vi "CMD_TRANSFORMG2L.vi"(8 "error in (no error)":errorcluster, 10 "Arguments":string[](array[string]), 11 "gScript Interpreter in":refnum<class "gScript Interpreter.lvclass">) -> (0 "error out":errorcluster, 3 "gScript Interpreter out":refnum<class "gScript Interpreter.lvclass">)   [LabVIEW 2017, in "gScript Interpreter.lvclass"]
uses:
  gScript Interpreter.lvclass
  Shared Components/Utils/Type Definitions/Position_Orientation.ctl
  Shared Components/Vec3d Class/Vec3d.lvclass
  Shared Components/Orient3d Class/Orient3d.lvclass
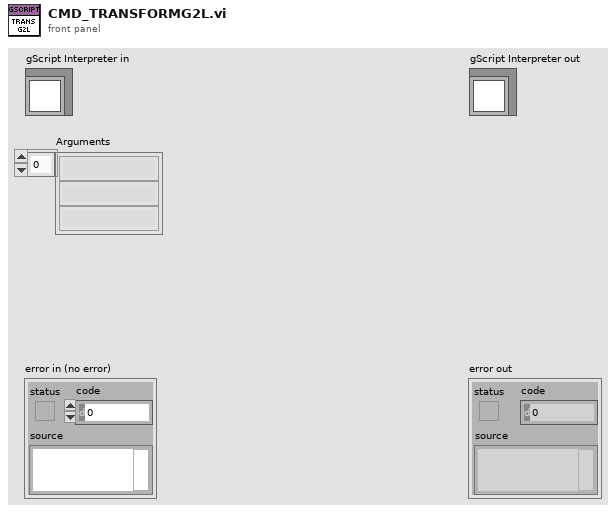
[diagram p1: front panel]
types:
  T1 = typedef "Position_Orientation.ctl" = cluster{"Center":refnum<class "Vec3d.lvclass">, "Orientation":refnum<class "Orient3d.lvclass">}
  T2 = typedef "Memory Cell.ctl" = cluster{"type":T3, "x":dbl, "y":dbl, "z":dbl, "w":dbl}
  T3 = typedef "Memory Cell Type Enum.ctl" = enum16{"integer", "float", "vector", "rotation"}
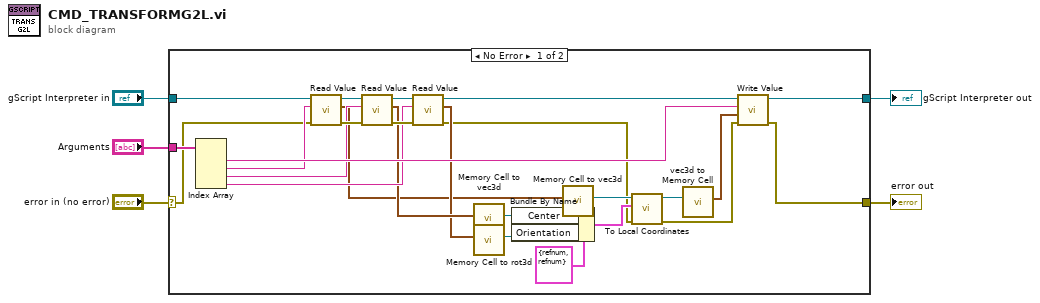
[diagram p0: block diagram]
diagram:
  n1 = case shown="No Error" "error in (no error)" {
    selector: "error in (no error)" -> [w25 w33]
    tunnel: [w28 w33] -> w4
    tunnel: [w29 w32] -> w2
    tunnel: "gScript Interpreter in" -> [w26 w32]
    tunnel: "Arguments" -> [w31 _]
    frame No Error {
      n2 = Index Array(array=w31) -> (element #1=w30:string, element #2=w27:string, element #3=w20:string, element #4=w19:string)  [unwired: 4 in]
      n3 = call-dynamic "Read Value.vi"("error in (no error)"=w25, "String in"=w27, "gScript Interpreter in"=w26) -> ("error out"=w22:errorcluster, "Memory Cell"=w12:T2, "gScript Interpreter out"=w24:refnum<class "gScript Interpreter.lvclass">)  [unwired: 6 in]
      n4 = call-dynamic "Read Value.vi"("error in (no error)"=w22, "String in"=w20, "gScript Interpreter in"=w24) -> ("error out"=w21:errorcluster, "Memory Cell"=w15:T2, "gScript Interpreter out"=w23:refnum<class "gScript Interpreter.lvclass">)  [unwired: 6 in]
      n5 = call-dynamic "Read Value.vi"("error in (no error)"=w21, "String in"=w19, "gScript Interpreter in"=w23) -> ("error out"=w10:errorcluster, "Memory Cell"=w14:T2, "gScript Interpreter out"=w9:refnum<class "gScript Interpreter.lvclass">)  [unwired: 6 in]
      n6 = call "Memory Cell to vec3d.vi"("Memory Cell"=w15) -> ("Vec3d out"=w17:refnum<class "Vec3d.lvclass">)  [unwired: 10 in]
      n7 = call "Memory Cell to rot3d.vi"("Memory Cell"=w14) -> ("Orient3d out"=w16:refnum<class "Orient3d.lvclass">)  [unwired: 10 in]
      n8 = Bundle By Name(cluster=T1 {"Center"=refnum, "Orientation"=refnum} ("Center/Orientation"), "Center"=w17, "Orientation"=w16) -> (w13:T1)
      n9 = call "Memory Cell to vec3d.vi"("Memory Cell"=w12) -> ("Vec3d out"=w11:refnum<class "Vec3d.lvclass">)  [unwired: 10 in]
      n10 = call "To Local Coordinates.vi"("error in"=w10, "Center/Orientation"=w13, "Global Coordinates"=w11) -> ("error out"=w6:errorcluster, "Local Coordinates"=w8:refnum<class "Vec3d.lvclass">)  [unwired: 7 in]
      n11 = call "vec3d to Memory Cell.vi"("Vec3d in"=w8) -> ("Memory Cell"=w7:T2)  [unwired: 10 in]
      n12 = call-dynamic "Write Value.vi"("error in (no error)"=w6, "Value"=w7, "Address"=w30, "gScript Interpreter in"=w9) -> ("error out"=w28:errorcluster, "gScript Interpreter out"=w29:refnum<class "gScript Interpreter.lvclass">)  [unwired: 6 in]
    }
    frame Error {
    }
  }
  "error out" <- w4
  "gScript Interpreter out" <- w2
